vi "Trace_Variables.vi"(0 "data_12_bit":u16[](array[numeric]), 1 "peakThreshold":u16, 2 "traceLength":i32, 3 "baselineThreshold":u16, 4 "Baseline":i16) -> (5 "return type":i32, 6 "properties":T1)   [LabVIEW 2013]
doc: "<B>Explanation of params</B>\nA description is included at the bottom.\n<B>uint16_t data_12_bit</B>: Array which holds event data\n<B>int16_t PeakThreshold</B>: This value is used to calculated the number of postive pulses and\n indicates when a pulse starts i.e. what the distance from a single point to the\n baseline should be before its called a pulse. This also applies to the end of a\n pulse i.e. the distance from the top of a pulse should be bigger than this value\n before its called a pulse, so a single 'pulse base' with two separate, high\n enough 'pulse heads' is still counted as two pulses.\n<B>const int32_t traceLength</B>: The length of the event data array\n<B>const uint16_t baselineThreshold</B>: This threshold determines when a single element is no longer\n part of the <B>Baseline</B> (note: this value is not linked to PeakThreshold). Using\n this value, the peak integral and cutoffs are calculated\n<B>const int16_t Baseline</B>: All calculation preformed here are with respect to this value\n<B>struct traceProperties *properties</B>: This struct, represented by a cluster in labview, holds all trace\n properties which are calculated using this node\n<B>int32_t traceVariables</B>: The return type for this function is always 0 (zero), because the fact that the\n baseline returns <B>-999</B> already indicates the occurence of an error\n\n<B>Contents of traceProperties struct</B>\nThis is also the sequence in which LABVIEW returns the cluster.\nstruct traceProperties\n{\n int16_t numberOfPeaks; // The number of positive pulses (peaks over <B>peakThreshold</B>)\n int16_t leftCutOff; // The element from the left which determines the front cutoff i.e. first element bigger than <B>baselineThreshold</B>, this can be a negative pulse!*\n int16_t rightCutOff; // The element from the left which determines the rear cutoff i.e. first element after last pulse, this can be a negative pulse!*\n int16_t pulseHeight; // The highest value found in the <B>data_12_bit</B> array\n int32_t pulseIntegral; // The sum of all elements not part of the baseline (> <B>baselineThreshold</B>)\n};\n* in order to calculate the baseline even after data reduction, we include some extra elements in the left and right cutoff (default is <B>25</B> extra elements)\n\n<B>Description</B>:\nThe code consists of a for loop which, if the basline is not <B>-999</B>, iterates over every element of the <B>data_12_bit</B> array. For every element it first substracts the baseline then it determines the highest element the number of pulses by using the <B>peakThreshold</B>, the pulse integral and both cutoffs are then calculated using the <B>baselineThreshold</B>."
uses:
  dll/Baseline.dll
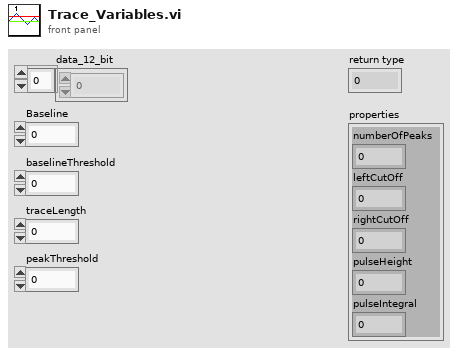
[diagram p1: front panel]
types:
  T1 = cluster{"numberOfPeaks":i16, "leftCutOff":i16, "rightCutOff":i16, "pulseHeight":i16, "pulseIntegral":i32}
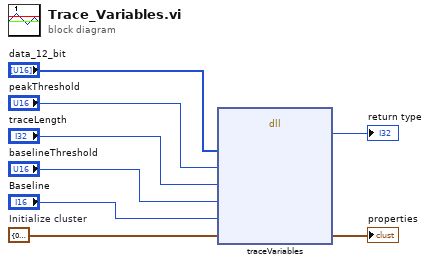
[diagram p0: block diagram]
diagram:
  w8 = T1 {"numberOfPeaks"=0, "leftCutOff"=0, "rightCutOff"=0, "pulseHeight"=0, "pulseIntegral"=0}  # Initialize cluster
  n1 = dll-call lib="C:/Users/SuperUser/Documents/HiSparc/HISPARC_baseline/VI/dll/Baseline.dll" fn="traceVariables"("data_12_bit"="data_12_bit", "peakThreshold"="peakThreshold", "traceLength"="traceLength", "baselineThreshold"="baselineThreshold", "Baseline"="Baseline", "properties"=w8) -> ("return type"=→"return type":i32, "properties"=→"properties":T1)  [unwired: 8 in, 2 out]
